vi "uTTA_Scale_ADC_Data.vi"(4 "Offset Voltage":dbl format="%.3pV", 5 "ADC Value":i32, 6 "PGA Setting":i32 min=0 max=3, 7 "Calibration":T1) -> (3 "Scaled Output":dbl)   [LabVIEW 2021]
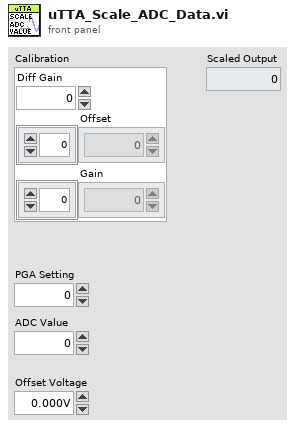
[diagram p1: front panel]
types:
  T1 = cluster{"Diff Gain":dbl, "Offset":dbl[], "Gain":dbl[]}
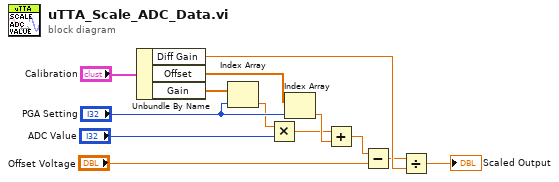
[diagram p0: block diagram]
diagram:
  n1 = Unbundle By Name("Calibration") -> ("Diff Gain"=w12:dbl, "Offset"=w10:dbl[], "Gain"=w9:dbl[])
  n2 = Index Array(array=w9, index="PGA Setting") -> (element=w6:dbl)
  n3 = Multiply(x=w6, y="ADC Value") -> (x*y=w4:dbl)
  n4 = Index Array(array=w10, index="PGA Setting") -> (element=w5:dbl)
  n5 = Add(x=w4, y=w5) -> (x+y=w3:dbl)
  n6 = Subtract(x=w3, y="Offset Voltage") -> (x-y=w1:dbl)
  n7 = Divide(x=w1, y=w12) -> (x/y=→"Scaled Output":dbl)
